vi "Kxx_Kxy_B_cs580 _KEguard2.vi"() -> ()   [LabVIEW 2023]
uses:
  <instrlib>/Keithley 622x LV 2009/Utility/Typedefs/KE622x -- Instrument Type.ctl
  Typedefs/Kxx_Kxy_state_machine_cases.ctl
  Z:/Labview Control Software/Keithley 622x LV 2009/Typedefs/KE622x -- On Off Control.ctl
  Z:/Labview Control Software/Keithley 622x LV 2009/Configure/Output/Typedefs/KE6221 -- Output Response.ctl
  Z:/Labview Control Software/Keithley 622x LV 2009/Configure/Source/Typedefs/KE622x -- Voltage Limit.ctl
  <vilib>/Analysis/1siggen.llb/Ramp Pattern by Samples.vi
  <vilib>/Analysis/baseanly.llb/Mean (DBL).vi
  <vilib>/Instr/_visa.llb/VISA Configure Serial Port (Instr).vi
  <vilib>/Utility/file.llb/Write To Spreadsheet File (string).vi
  MQM Data Transfer All.vi
  <vilib>/Utility/file.llb/Read Delimited Spreadsheet (DBL).vi
  Global Variables/Thermometers.vi
  <instrlib>/Keithley 622x LV 2009/Keithley 622x.lvlib
  <vilib>/Analysis/NI_AALBase.lvlib
  Drivers/Keithley 2182/Keithley 2182.lvlib
panel:
  in  "Kxy data":dbl[](array[numeric])
  in  "Kxx data":dbl[](array[numeric])
  in  "T_avg data":dbl[](array[numeric])
  in  "dTxx":dbl
  in  "HTR Power":dbl
  in  "dTxy":dbl
  in  "T_avg":dbl
  in  "T_H Array":dbl[](array[numeric])
  in  "T_C1 Array":dbl[](array[numeric])
  in  "T_C2 Array":dbl[](array[numeric])
  in  "HTR Voltage Array":dbl[](array[numeric])
  in  "?":enum32{"Setup", "Plotting", "Error Readouts"}(tab)
  in  "DeltaT (fraction of tsp)":dbl=0.05
  in  "Sample_t":dbl
  in  "Sample_w":dbl
  in  "Sample_Lxx":dbl
  in  "Heater Current File (H, T, current)":path
  out "Heater Current \nArray":dbl[](array[numeric])
  out "Ramp Pattern":dbl[](array[numeric])
  in  "Tstart (K)":dbl=3.0
  in  "Tend (K)":dbl=4.0
  in  "Steps":i16=2
  in  "Log (on)\nLin (off) (Temperature setpoints)":bool=TRUE
  in  "Initial Heater Current (A)":dbl=1e-06
  in  "Hstart (Oe)":dbl
  in  "Hend (Oe)":dbl
  in  "Field Steps":i16=1
  in  "Log (on)\nLin (off)  (Field setpoints)":bool
  in  "Sample_Lxy":dbl=0.0005
  in  "Test?":bool
  in  "Calibration Only?":bool
  in  "Exchange gas?":bool
  in  "Preset Heater Current Array?":bool
  in  "T Current Source":refnum<visa-resource-name>="6221B"
  in  "HTR Current Source":refnum<visa-resource-name>="CS580-1"
  in  "DC Voltmeter":refnum<visa-resource-name>="2182"
  in  "Thermometer Frequency (Hz)":string="37"
  in  "Initial Thermometer Current (A)":string="1.4142e-7"
  in  "Final Field (Oe)":dbl
  in  "Final Temperature (K)":dbl=1.7
  in  "Filename":path=path "C:/User Data/Luke/Kxx/NaYSe2/NaYSe2_1p7_100K_log_100_9T_8_23_21"
  in  "Heater Only?":bool
  in  "Running avg size":dbl=500.0 format="%#_13g"
  in  "std/mean thresh":dbl=1e-05 format="%#_13g"
  in  "slope/mean thresh":dbl=1e-07 format="%#_13g"
  in  "Guard HTR Current Source":refnum<visa-resource-name>
  in  "HTR Guard Current Factor":dbl
  out "Kxx Plot":cluster{dbl[], dbl[]}(graph)
  out "Kxy Plot":cluster{dbl[], dbl[]}(graph)
  out "All Data":cluster{dbl[], dbl[]}[](graph)
  in  "Finish":bool
  out "Data Rate (ms)":u32
  in  "Delay (ms)":dbl=300.0
  in  "Quick Data Recording":bool=TRUE
  out "Tsp":dbl
  out "HTR_Current":dbl
  out "Mask":dbl
  out "HTR_Voltage":dbl
  out "T_H":dbl
  out "T_C1":dbl
  out "I_therm":dbl
  out "T_C2":dbl
  in  "Display Elements":cluster{"X":bool, "Y":bool, "Name":u16}[](array[cluster]) {"Name" items=["Time (ms)", "Temperature (K)", "Field (T)", "LI_1_X", "LI_1_theta", "LI_2_X", "LI_2_theta", "LI_3_X", "LI_3_theta", "DC_V", "DC_I", "mask", "tsp", "I_therm", "T_H", "T_C1", "T_C2", "Fieldsp"]}
  in  "X-Axis":u16(ring) items=["Linear", "Reciprocal", "Log10"]
  in  "Y-Axis":u16(ring) items=["Linear", "Reciprocal", "Log10"]
  out "Fieldsp":dbl
  out "Global Stop":bool
  out "Thermometers":cluster{"T_H":dbl, "T_C1":dbl, "T_C2":dbl}
  out "QD error out":errorcluster
  out "KE6221 error out":errorcluster
  out "KE2182 error out":errorcluster
  out "Guard Heater Error":errorcluster
  # "TURN ON HIGH VACUUM!"
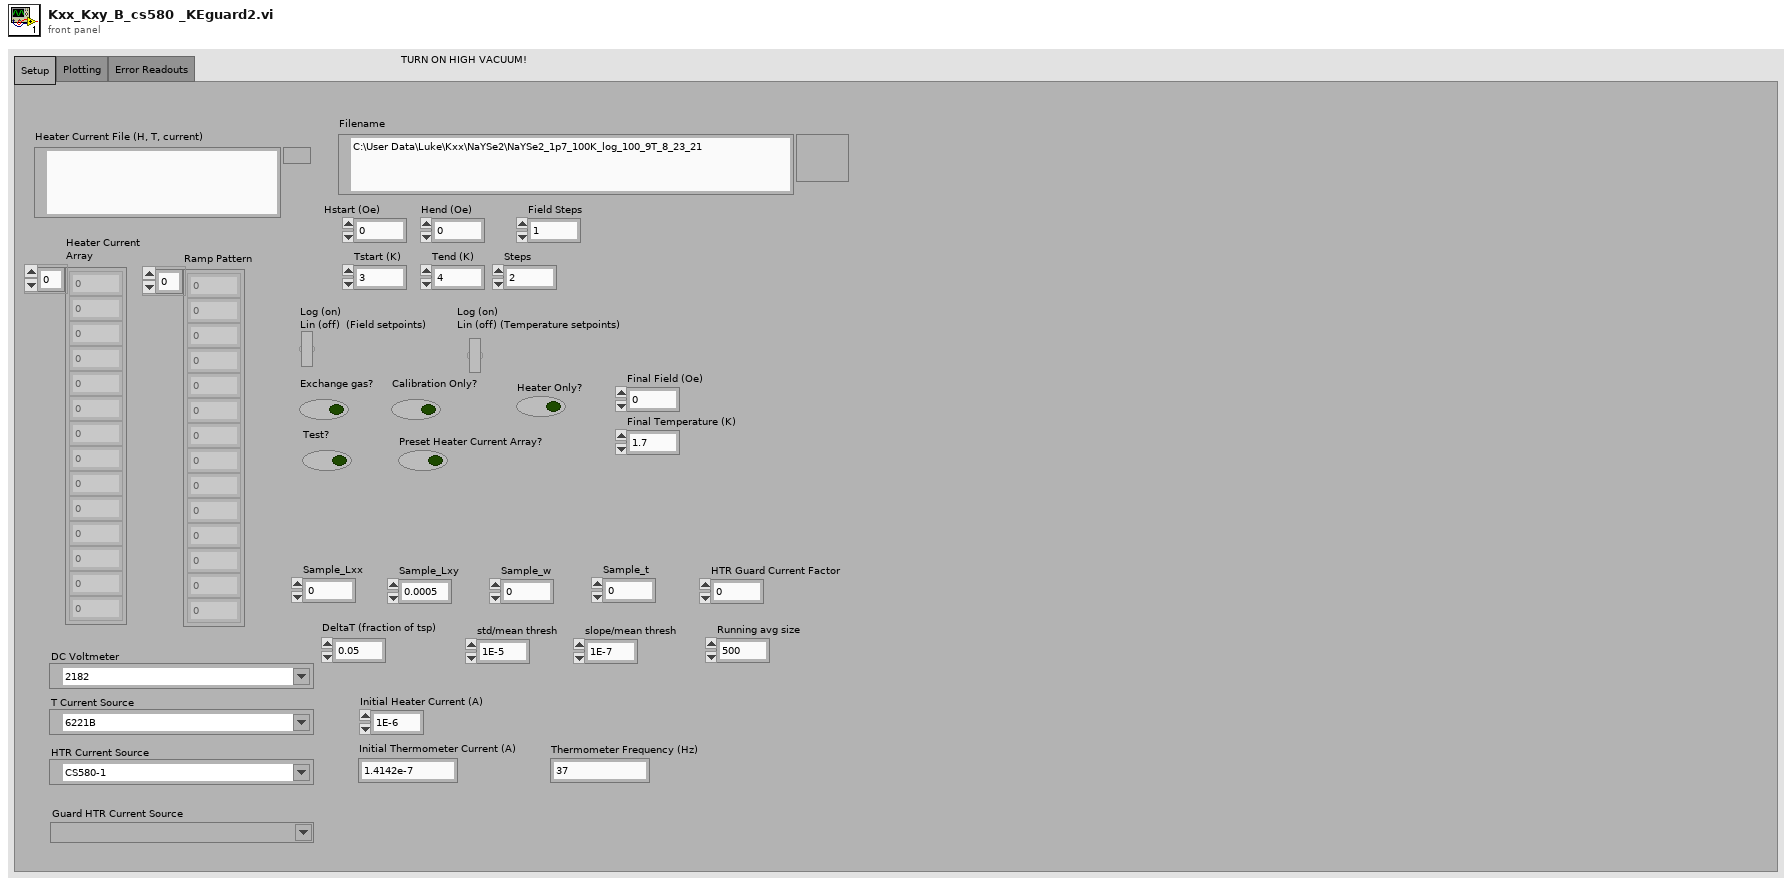
[diagram p1: front panel]
types:
  T1 = typedef "Keithley 622x.lvlib/KE622x -- Instrument Type.ctl" = enum16{"KE6220", "KE6221"}
  T2 = typedef "Kxx_Kxy_state_machine_cases.ctl" = enum16{"Initialize", "Wait to Stabilize (no heat)", "Measure (no heat)", "Turn on Heater, stabilize", "Measure (heat)", "Turn off Heater", "Assign Heater Current", "Plot", "End"}
  T3 = typedef "Keithley 622x.lvlib/KE622x -- Voltage Limit.ctl" = dbl
  T4 = typedef "Keithley 622x.lvlib/KE6221 -- Output Response.ctl" = enum16{"Fast", "Slow"}
  T5 = typedef "Keithley 622x.lvlib/KE622x -- On Off Control.ctl" = enum16{"Off", "On"}
  T6 = cluster{"T_avg data":dbl[], "Kxx data":dbl[], "Kxy data":dbl[]}
  T7 = cluster{"T_avg":dbl, "dTxx":dbl, "dTxy":dbl, "HTR Power":dbl, "HTR Voltage Array":dbl[], "T_H Array":dbl[], "T_C1 Array":dbl[], "T_C2 Array":dbl[], "error out":errorcluster}
  T8 = typedef "ZI_Frontpanel_All.ctl" = cluster{"Lockin 1 Demod 0":cluster{"R(V)":dbl, "Theta (deg)":dbl, "Timestamp (ms)":u32, "X(V)":dbl, "Y(V)":dbl, "frequency (Hz)":dbl, "output voltage (V)":dbl}, "Lockin 2 Demod 0":cluster{"R(V)":dbl, "Theta (deg)":dbl, "Timestamp (ms)":u32, "X(V)":dbl, "Y(V)":dbl, "frequency (Hz)":dbl, "output voltage (V)":dbl}, "Lockin 3 Demod 0":cluster{"R(V)":dbl, "Theta (deg)":dbl, "Timestamp (ms)":u32, "X(V)":dbl, "Y(V)":dbl, "frequency (Hz)":dbl, "output voltage (V)":dbl}, "Lockin 4 Demod 0":cluster{"R(V)":dbl, "Theta (deg)":dbl, "Timestamp (ms)":u32, "X(V)":dbl, "Y(V)":dbl, "frequency (Hz)":dbl, "output voltage (V)":dbl}, "LI1 active":bool, "LI2 active":bool, "LI3 active":bool, "LI4 active":bool}
  T9 = typedef "PPMS_Status.ctl" = cluster{"Field":cluster{"Field (T)":dbl, "Field stable":bool, "Timestamp (ms)":u32}, "Temperature":cluster{"Temperature (K)":dbl, "Temperature stable":bool, "Timestamp (ms)":u32}}
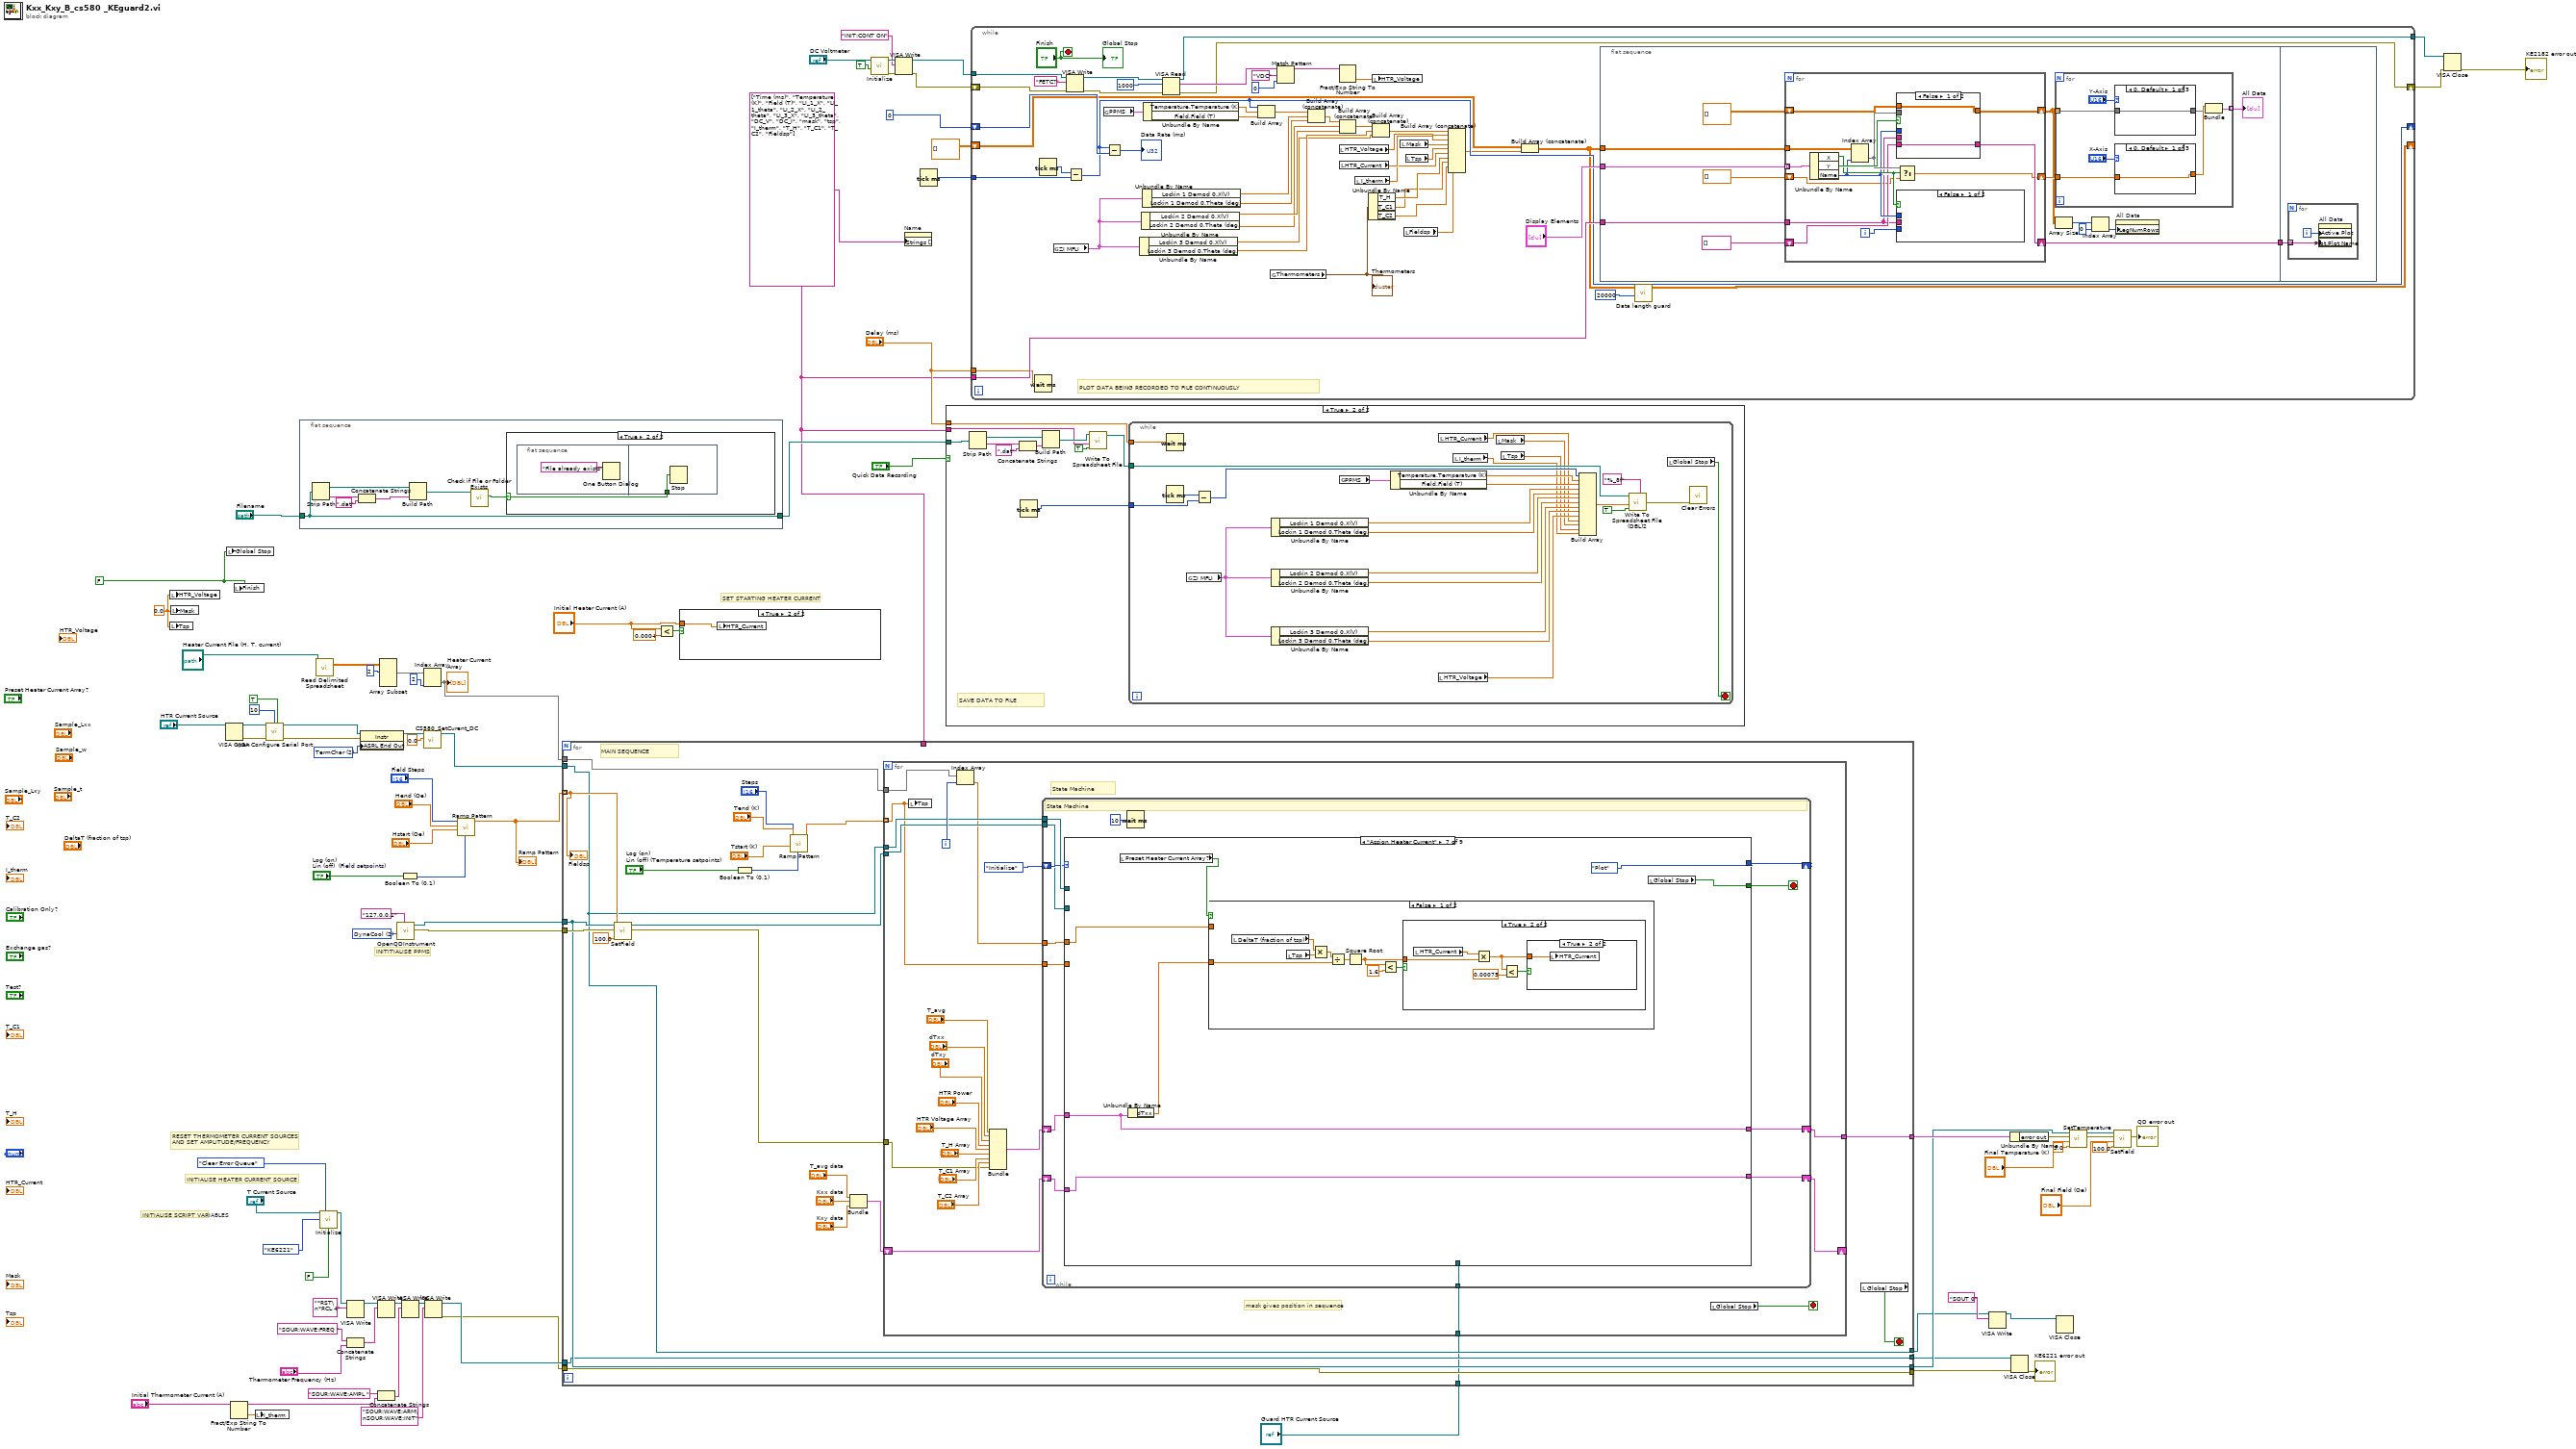
[diagram p0: block diagram]
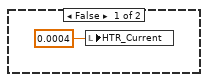
[diagram p2: hidden frame]
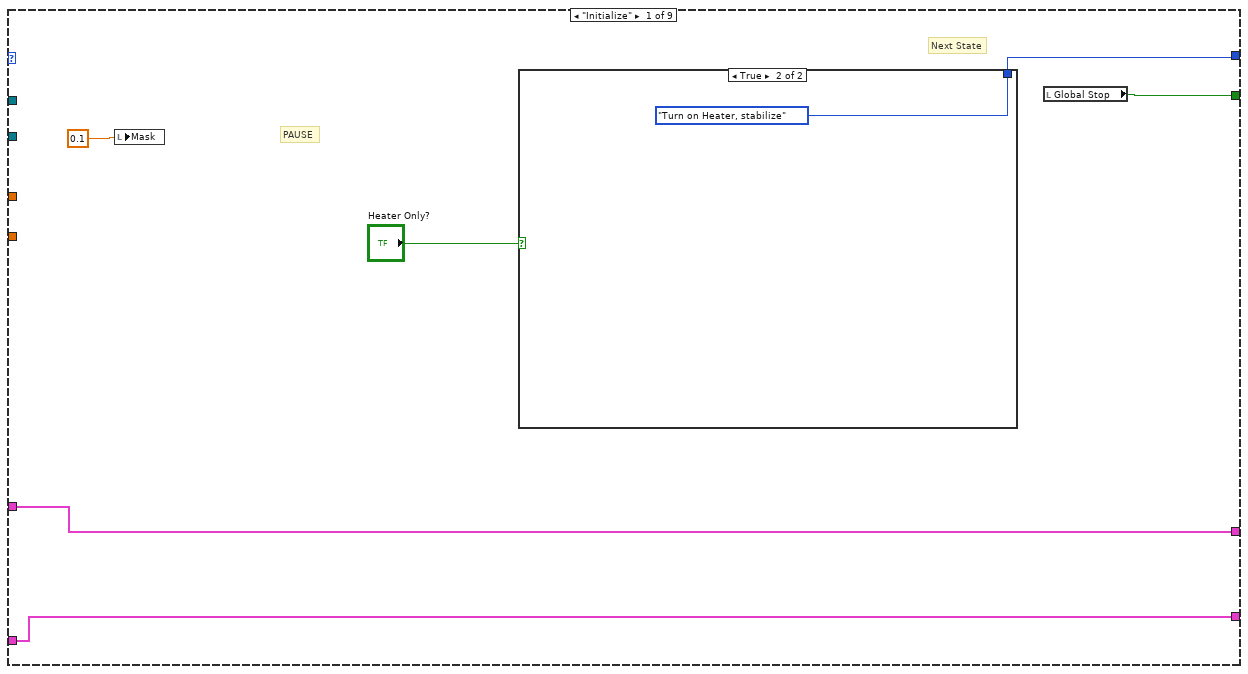
[diagram p4: hidden frame]
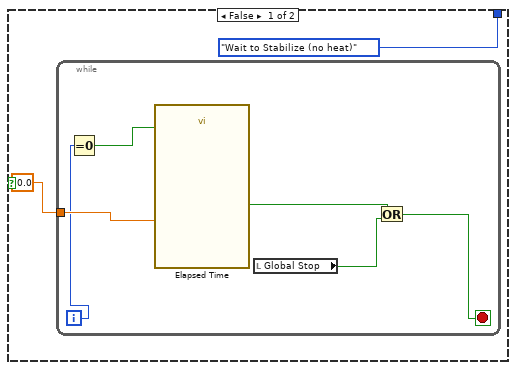
[diagram p5: hidden frame]
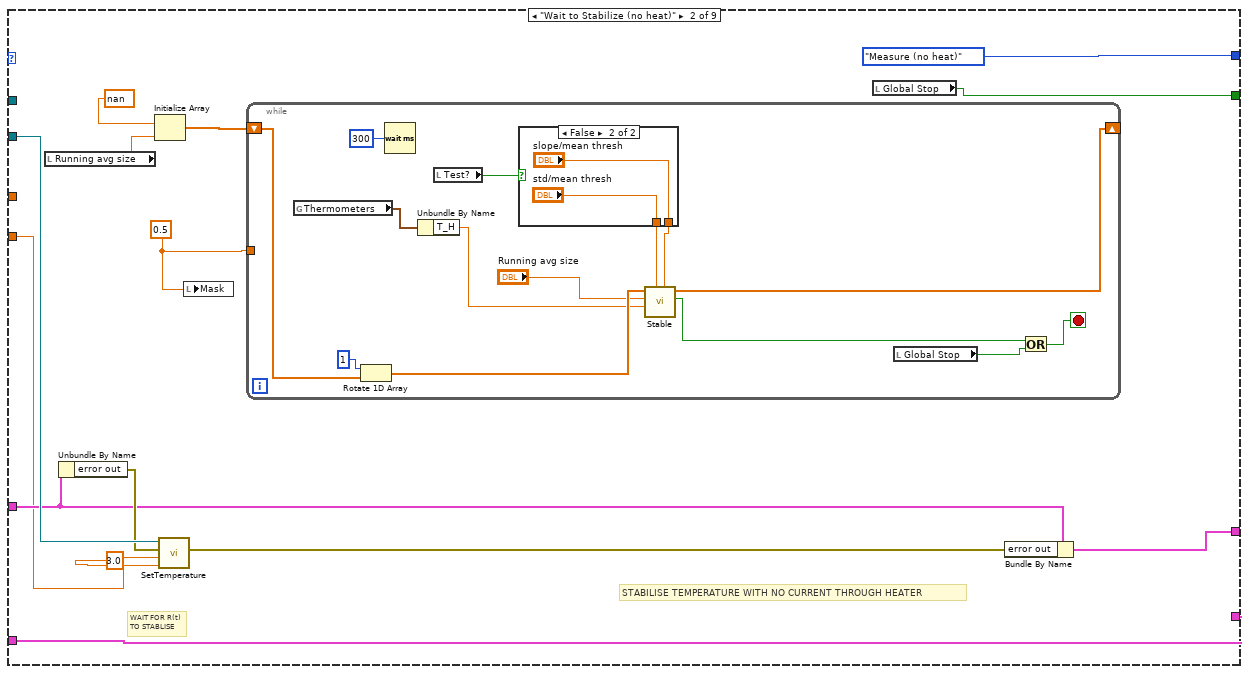
[diagram p6: hidden frame]
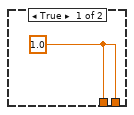
[diagram p7: hidden frame]
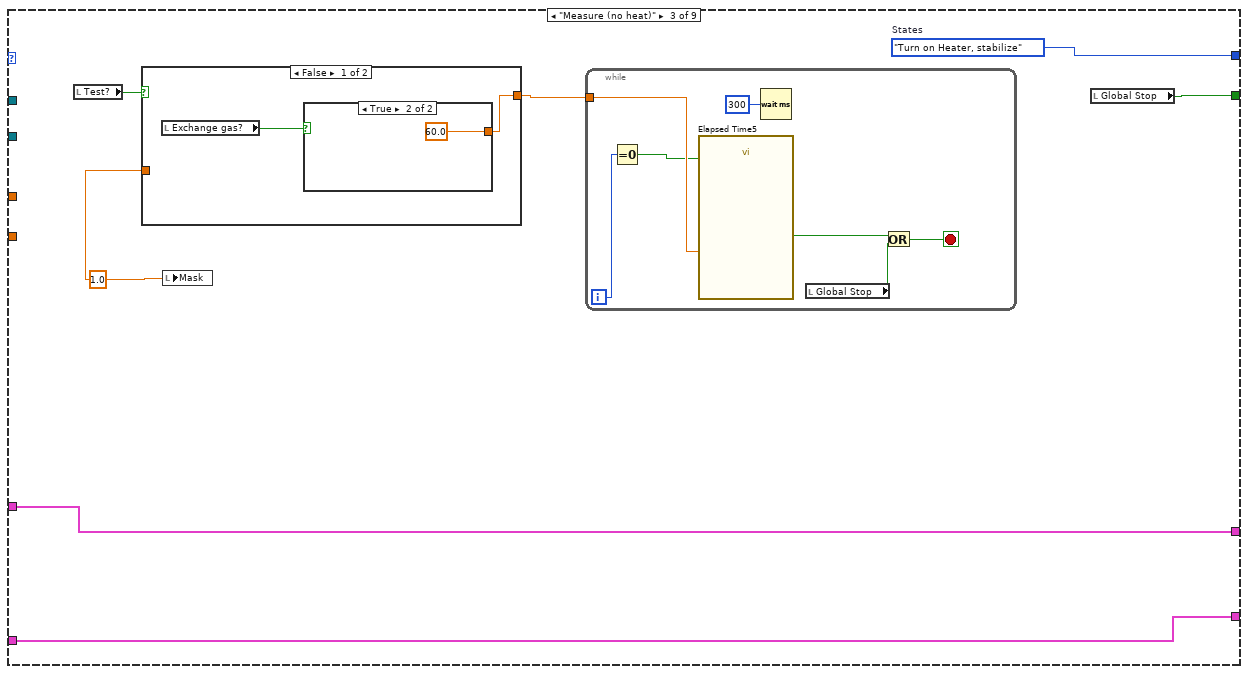
[diagram p8: hidden frame]
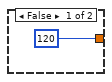
[diagram p9: hidden frame]
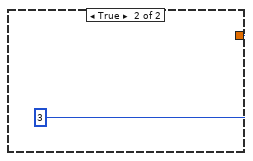
[diagram p10: hidden frame]
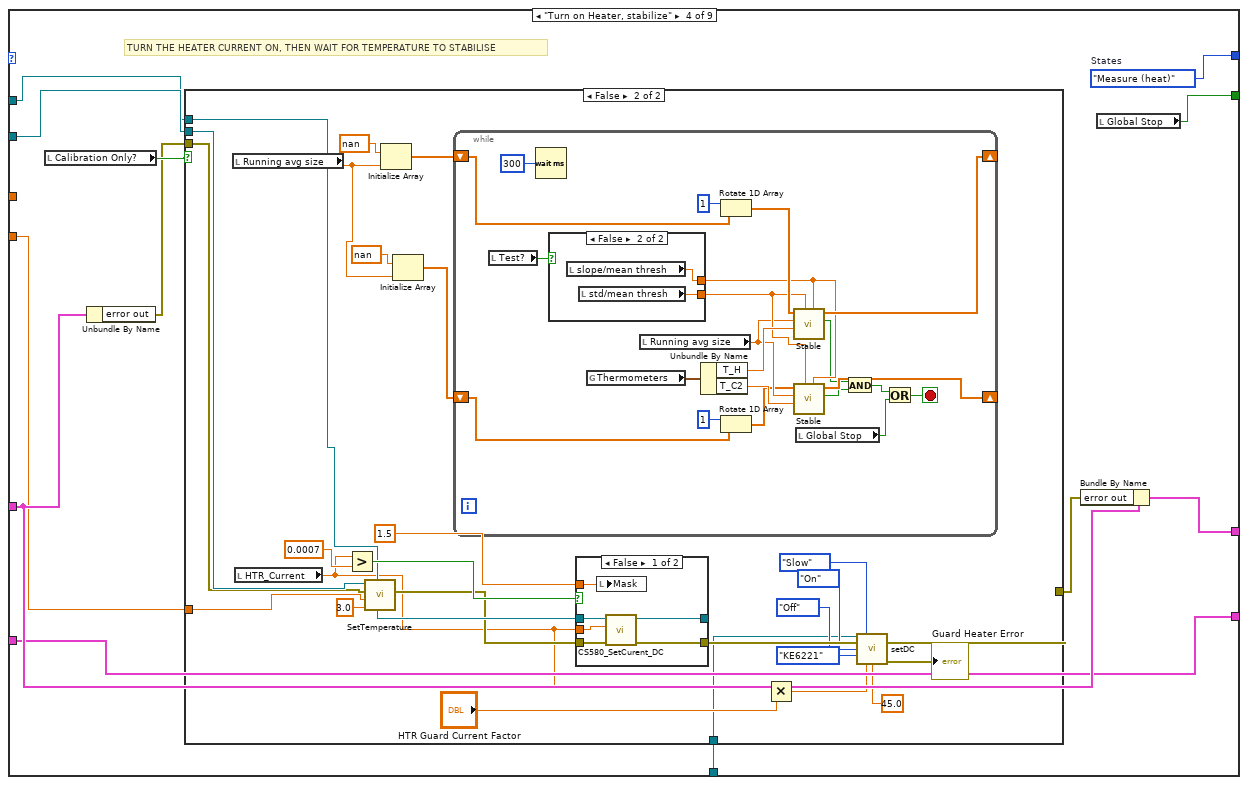
[diagram p11: hidden frame]
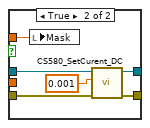
[diagram p13: hidden frame]
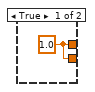
[diagram p14: hidden frame]
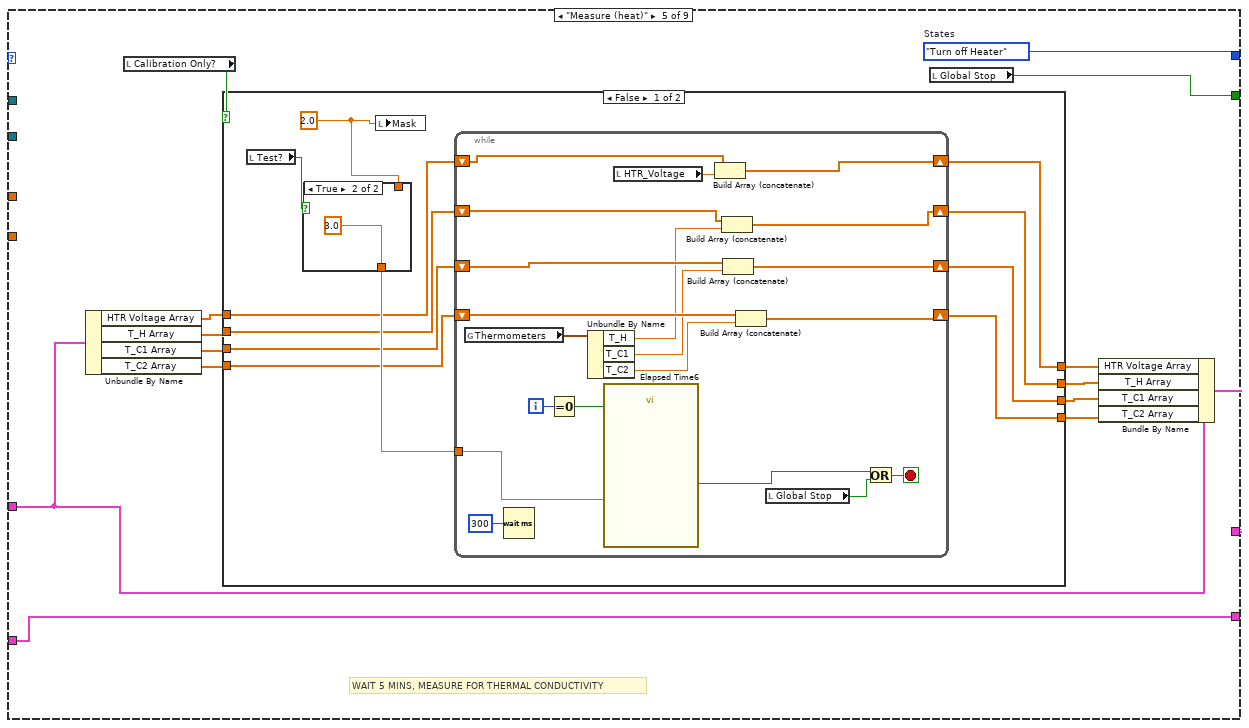
[diagram p15: hidden frame]
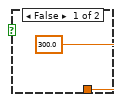
[diagram p16: hidden frame]
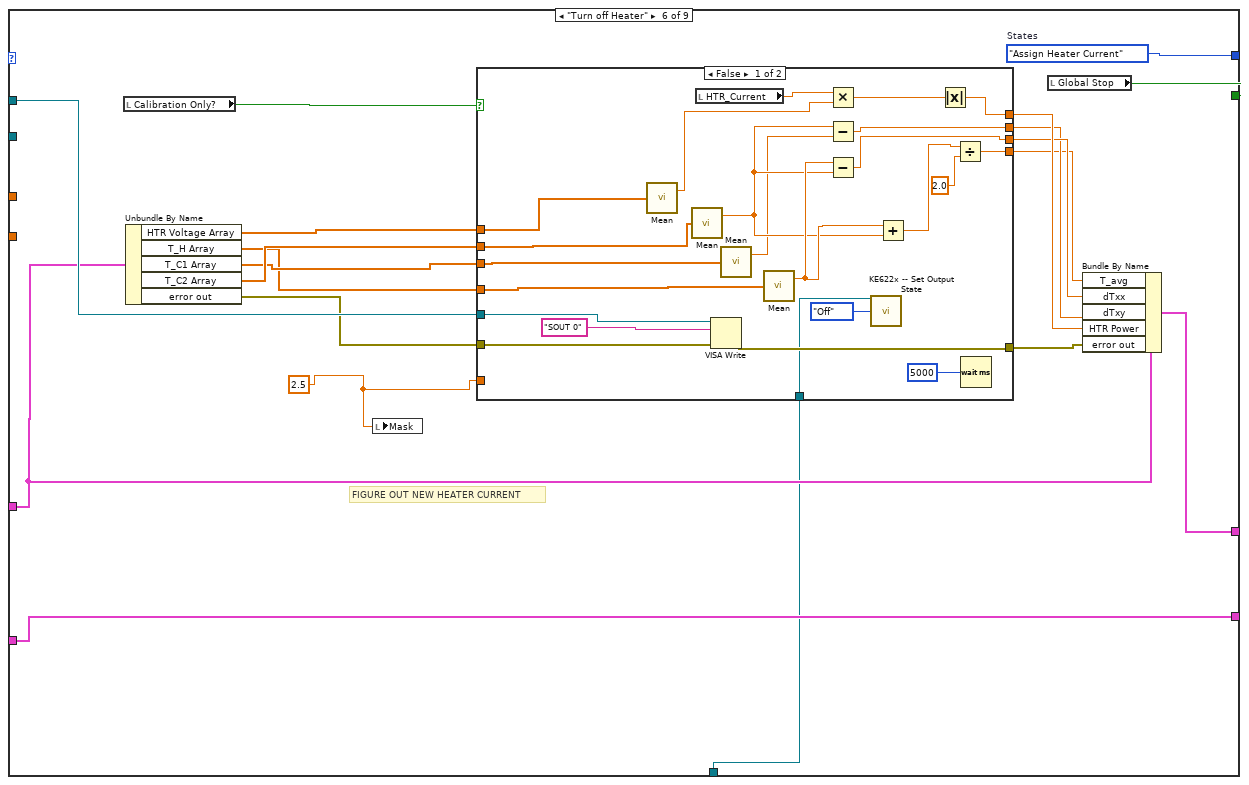
[diagram p18: hidden frame]
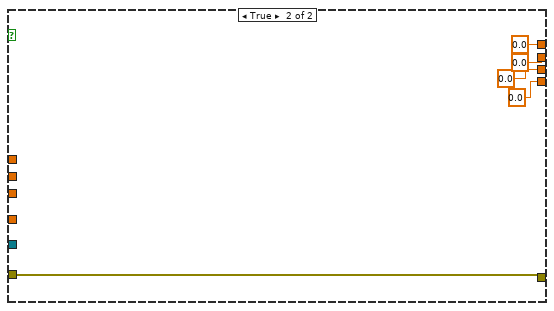
[diagram p19: hidden frame]
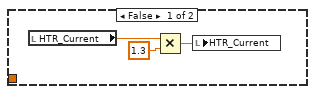
[diagram p20: hidden frame]
diagram:
  w7 = FALSE ("Calibration confirmed")
  w6 = string[] ["Time (ms)", "Temperature (K)", "Field (T)", "LI_1_X", "LI_1_theta", "LI_2_X", "LI_2_theta", "LI_3_X", "LI_3_theta", "DC_V", "DC_I", "mask", "tsp", "I_therm", "T_H", "T_C1", "T_C2", "Fieldsp"] ("element")
  w57 = u16 2 items=["None", "Last Bit", "TermChar", "Break"] ("Serial Settings:End Mode for Writes")
  w75 = 0.0 ("Mask")
  w82 = 2 items=["PPMS", "VersaLab", "DynaCool", "SVSM"] ("Instrument Type")
  # "SET STARTING HEATER CURRENT"
  # "INITIALISE HEATER CURRENT SOURCE"
  # "RESET THERMOMETER CURRENT SOURCES\nAND SET AMPLITUDE/FREQUENCY"
  # "INITITIALISE PPMS"
  # "INITIALISE SCRIPT VARIABLES"
  n1 = local write "HTR_Voltage"(w75) -> ()
  n2 = local write "Tsp"(w75) -> ()
  n3 = local write "Mask"(w75) -> ()
  n4 = VISA Open(VISA resource name="HTR Current Source") -> (VISA resource name=w53:refnum<visa-resource-name>, error out=w54:errorcluster)  [unwired: 4 in]
  n5 = local write "Global Stop"(w7) -> ()
  n6 = Fract/Exp String To Number(string="Initial Thermometer Current (A)") -> (number=w65:dbl)  [unwired: 3 in, 1 out]
  n7 = local write "Finish"(w7) -> ()
  n8 = local write "I_therm"(w65) -> ()
  n9 = call-poly "VISA Configure Serial Port"("VISA resource name"=w53, "termination char\n(0xA = '\\n' = LF)"=u8 10 ("termination char\n(0xA = '\\n' = LF)"), "Enable Termination\nChar (T)"=TRUE ("Enable Termination\nChar (T)"), "error in (no error)"=w54) -> ("VISA resource name out"=w55:refnum<visa-resource-name>, "error out"=w56:errorcluster)  [unwired: 10 in]
  n10 = flat-sequence {
    tunnel: "Filename" -> [w89]
    tunnel: [w89] -> w26
    frame #0 {
      n11 = Strip Path(path=w89) -> (stripped path=w93:path, name=w90:string)
      n12 = Concatenate Strings(w90, ".dat") -> (w92:string)
      n13 = Build Path(base path=w93, name or relative path=w92) -> (appended path=w88:path)
      n14 = call <vilib>:"Check if File or Folder Exists.vi"("path"=w88) -> ("file or folder exists?"=w87:bool)  [unwired: 8 in, 2 out]
      n15 = case shown="True" w87 {
        selector: w87 -> [_ w94]
        frame False {
        }
        frame True {
          n16 = flat-sequence {
            tunnel: w94 -> [w96]
            frame #0 {
              n17 = One Button Dialog(message="File already exists") -> ()  [unwired: 1 in, 1 out]
            }
            frame #1 {
              n18 = Stop(stop? (T)=w96) -> ()
            }
          }
        }
      }
    }
  }
  n19 = call-poly <vilib>:"Read Delimited Spreadsheet.vi"("file path (dialog if empty)"="Heater Current File (H, T, current)") -> ("all rows"=w48:dbl[][])  [unwired: 9 in, 5 out]
  n20 = call <instrlib>:"Initialize.vi"("VISA resource name"="T Current Source", "Error Queue Option"=enum16{"Clear Error Queue", "Error Query"}."Clear Error Queue", "Instrument Type"=KE622x_--_Instrument_Type."KE6221", "Reset? (T)"=FALSE) -> ("VISA resource name out"=w73:refnum<visa-resource-name>)  [unwired: 10 in, 1 out]
  n21 = VISA Write(VISA resource name=w73, write buffer="*RST\n*RCL 4") -> (VISA resource name out=w67:refnum<visa-resource-name>)  [unwired: 1 in, 2 out]
  n22 = Concatenate Strings("SOUR:WAVE:FREQ " ("string"), "Thermometer Frequency (Hz)") -> (w72:string)
  n23 = property class="Instr"(reference=w55, error in=w56, "ASRL End Out"=w57) -> (reference out=w51:refnum<visa-resource-name>)  [unwired: 1 out]
  n24 = VISA Write(VISA resource name=w67, write buffer=w72) -> (VISA resource name out=w66:refnum<visa-resource-name>)  [unwired: 1 in, 2 out]
  n25 = Concatenate Strings("SOUR:WAVE:AMPL " ("string"), "Initial Thermometer Current (A)") -> (w69:string)
  n26 = Array Subset(array=w48, index (row)=2 ("index")) -> (w46:dbl[][])  [unwired: 3 in]
  n27 = call <instrlib>:"OpenQDInstrument.vi"("IP Address"="127.0.0.1", "Instrument Type"=w82) -> ("error out"=w25:errorcluster, "Instrument Ref"=w23:refnum<k24>)  [unwired: 6 in]
  n28 = VISA Write(VISA resource name=w66, write buffer=w69) -> (VISA resource name out=w43:refnum<visa-resource-name>)  [unwired: 1 in, 2 out]
  n29 = Boolean To (0,1)(Boolean="Log (on)\nLin (off)  (Field setpoints)") -> (0, 1=w60:i16)
  n30 = Index Array(array=w46, index (col)=2 ("disabled index (col)")) -> (element=w41:dbl[])  [unwired: 1 in]
  "Heater Current \nArray" <- w41
  n31 = call "CS580_SetCurent_DC.vi"("Current (A)"=0.0, "VISA Refnum in"=w51) -> ("VISA resource name out"=w24:refnum<visa-resource-name>)  [unwired: 8 in, 1 out]
  n32 = VISA Write(VISA resource name=w43, write buffer="SOUR:WAVE:ARM\nSOUR:WAVE:INIT") -> (VISA resource name out=w16:refnum<visa-resource-name>, error out=w12:errorcluster)  [unwired: 1 in, 1 out]
  n33 = call-poly <vilib>:"Ramp Pattern.vi"("type"=w60, "start"="Hstart (Oe)", "end"="Hend (Oe)", "samples"="Field Steps") -> ("Ramp Pattern"=w42:dbl[])  [unwired: 6 in, 1 out]
  "Ramp Pattern" <- w42
  n34 = for {
    tunnel: w42 -> [w119] mode=indexing
    tunnel: w23 -> [w102]
    tunnel: w25 -> [w117]
    tunnel: w41 -> [w110]
    tunnel: w24 -> [w98]
    tunnel: [w103] -> w18
    tunnel: w16 -> [w101]
    tunnel: [w102] -> w15
    tunnel: [w101] -> w14
    tunnel: w12 -> [w100]
    tunnel: [w100] -> w11
    tunnel: [w98] -> w4
    tunnel: w6 -> [_]
    tunnel: "Guard HTR Current Source" -> [w97]
    stop <- w99 stop-if-true
    # "MAIN SEQUENCE"
    n35 = call <instrlib>:"SetField.vi"("Rate"=100.0, "Field"=w119, "error in (no error)"=w117, "Instrument Ref In"=w102) -> ("error out"=w109:errorcluster, "Instrument Ref Out"=w108:refnum<k24>)  [unwired: 3 in, 1 out]
    n36 = Boolean To (0,1)(Boolean="Log (on)\nLin (off) (Temperature setpoints)") -> (0, 1=w114:i16)
    n37 = call-poly <vilib>:"Ramp Pattern.vi"("type"=w114, "start"="Tstart (K)", "end"="Tend (K)", "samples"="Steps") -> ("Ramp Pattern"=w116:dbl[])  [unwired: 6 in, 1 out]
    n38 = Bundle("T_avg data"="T_avg data", "Kxx data"="Kxx data", "Kxy data"="Kxy data") -> (w104:T6)  [unwired: 1 in]
    n39 = for {
      tunnel: w116 -> [w123] mode=indexing
      tunnel: w110 -> [w141]
      tunnel: w109 -> [w128]
      tunnel: w98 -> [w138]
      tunnel: w108 -> [w137]
      shift-right: [w122] -> _
      shift-left: w104 -> [w121]
      tunnel: [w125] -> w103
      tunnel: w97 -> [w120]
      i -> [w140]
      stop <- w124 stop-if-true
      # "State Machine"
      # "mask gives position in sequence"
      n40 = local write "Tsp"(w123) -> ()
      n41 = Index Array(array=w141, index=w140) -> (element=w126:dbl)
      n42 = Bundle("T_avg"="T_avg", "dTxx"="dTxx", "dTxy"="dTxy", "HTR Power"="HTR Power", "HTR Voltage Array"="HTR Voltage Array", "T_H Array"="T_H Array", "T_C1 Array"="T_C1 Array", "T_C2 Array"="T_C2 Array", "error out"=w128) -> (w127:T7)  [unwired: 1 in]
      n43 = while {
        shift-right: [w154] -> _
        shift-left: Kxx_Kxy_state_machine_cases."Initialize" -> [w151]
        tunnel: w138 -> [w152]
        tunnel: w137 -> [w147]
        shift-right: [w150] -> w125
        shift-left: w127 -> [w149]
        tunnel: w126 -> [w148]
        tunnel: w123 -> [w145]
        shift-right: [w144] -> w122
        shift-left: w121 -> [w143]
        tunnel: w120 -> [w142]
        stop <- w146 stop-if-true
        # "State Machine"
        n44 = case shown="\"Assign Heater Current\"" w151 {
          selector: w151 -> [_ _ _ _ _ _ _ _ w447]
          tunnel: w147 -> [_ w179 _ w230 _ _ _ _ _]
          tunnel: [w159 Kxx_Kxy_state_machine_cases."Measure (no heat)" w205 w228 w306 w361 Kxx_Kxy_state_machine_cases."Plot" w435 w447] -> w154
          tunnel: w152 -> [_ _ _ w229 _ w362 _ _ _]
          tunnel: [w158 w175 w204 w224 w297 w349 w396 w434 w446] -> w150
          tunnel: w149 -> [w158 w176 w204 w226 w296 w356 w396 w434 w446]
          tunnel: w143 -> [w157 w174 w203 w223 w295 w348 w395 w425 w445]
          tunnel: [w157 w174 w203 w223 w295 w348 w395 w421 w445] -> w144
          tunnel: w148 -> [_ _ _ _ _ _ w394 _ _]
          tunnel: [w156 w173 w202 w222 w294 w347 w393 w418 TRUE] -> w146
          tunnel: w145 -> [_ w172 _ w221 _ _ _ _ _]
          tunnel: w142 -> [_ _ _ w220 _ w345 _ _ _]
          frame "Initialize" {
            # "Next State"
            # "PAUSE"
            n45 = local write "Mask"(0.1 ("Mask")) -> ()
            n46 = case shown="True" "Heater Only?" {
              tunnel: [Kxx_Kxy_state_machine_cases."Wait to Stabilize (no heat)" Kxx_Kxy_state_machine_cases."Turn on Heater, stabilize"] -> w159
              frame False {
                n47 = while {
                  tunnel: 10.0 ("Time Target (s)") -> [w168]
                  i -> [w164]
                  stop <- w165 stop-if-true
                  n48 = Equal To 0?(x=w164) -> (x = 0?=w163:bool)
                  n49 = call "Elapsed Time"("Time Target (s)"=w168, "Reset"=w163) -> ("Time has Elapsed"=w167:bool)  [unwired: 10 in, 7 out]
                  n50 = local read "Global Stop"() -> (w166:bool)
                  n51 = Or(x=w167, y=w166) -> (x .or. y?=w165:bool)
                }
              }
              frame True {
              }
            }
            n52 = local read "Global Stop"() -> (w156:bool)
          }
          frame "Wait to Stabilize (no heat)" {
            w170 = 0.5 ("Mask")
            # "STABILISE TEMPERATURE WITH NO CURRENT THROUGH HEATER"
            # "WAIT FOR R(t)\nTO STABLISE"
            n53 = local read "Running avg size"() -> (w181:dbl)
            n54 = Unbundle By Name(w176) -> ("error out"=w177:errorcluster)
            n55 = Initialize Array(nan ("Element"), w181) -> (w183:dbl[])
            n56 = call <instrlib>:"SetTemperature.vi"("Rate"=3.0, "Temperature"=w172, "error in (no error)"=w177, "Instrument Ref In"=w179) -> ("error out"=w171:errorcluster)  [unwired: 3 in, 2 out]
            n57 = local write "Mask"(w170) -> ()
            n58 = while {
              shift-right: [w186] -> _
              shift-left: w183 -> [w196]
              tunnel: w170 -> [_]
              stop <- w192 stop-if-true
              n59 = global read "Thermometers.vi" "Thermometers"() -> (w191:cluster{"T_H":dbl, "T_C1":dbl, "T_C2":dbl})
              n60 = Rotate 1D Array(1:w196, 2:1 ("n")) -> (0:w190:dbl[])
              n61 = Wait (ms)(milliseconds to wait=u32 300) -> ()  [unwired: 1 out]
              n62 = Unbundle By Name(w191) -> ("T_H"=w188:dbl)
              n63 = local read "Test?"() -> (w194:bool)
              n64 = case shown="False" w194 {
                tunnel: [w198 "slope/mean thresh"] -> w187
                tunnel: [w198 "std/mean thresh"] -> w184
                frame True {
                  w198 = 1.0 ("y")
                }
                frame False {
                }
              }
              n65 = call "Stable.vi"("slope/mean thresh"=w187, "std/mean thresh"=w184, "New data point"=w188, "Number of points"="Running avg size", "Array in"=w190) -> ("Stable?"=w185:bool, "Array out"=w186:dbl[])  [unwired: 5 in]
              n66 = local read "Global Stop"() -> (w193:bool)
              n67 = Or(x=w185, y=w193) -> (x .or. y?=w192:bool)
            }
            n68 = local read "Global Stop"() -> (w173:bool)
            n69 = Bundle By Name(cluster=w176, "error out"=w171) -> (w175:T7)
          }
          frame "Measure (no heat)" {
            w205 = Kxx_Kxy_state_machine_cases."Turn on Heater, stabilize"  # States
            w201 = 1.0 ("Mask")
            n70 = local read "Test?"() -> (w207:bool)
            n71 = case shown="False" w207 {
              tunnel: [w208 u32 3 ("milliseconds to wait")] -> w206
              tunnel: w201 -> [_ _]
              frame False {
                n72 = local read "Exchange gas?"() -> (w209:bool)
                n73 = case shown="True" w209 {
                  tunnel: [120 60.0 ("Time to Wait (s)")] -> w208
                  frame False {
                  }
                  frame True {
                  }
                }
              }
              frame True {
              }
            }
            n74 = local write "Mask"(w201) -> ()
            n75 = while {
              tunnel: w206 -> [w217]
              i -> [w214]
              stop <- w216 stop-if-true
              n76 = Equal To 0?(x=w214) -> (x = 0?=w213:bool)
              n77 = call "Elapsed Time5"("Time Target (s)"=w217, "Reset"=w213) -> ("Time has Elapsed"=w215:bool)  [unwired: 10 in, 7 out]
              n78 = Wait (ms)(milliseconds to wait=u32 300) -> ()  [unwired: 1 out]
              n79 = local read "Global Stop"() -> (w219:bool)
              n80 = Or(x=w215, y=w219) -> (x .or. y?=w216:bool)
            }
            n81 = local read "Global Stop"() -> (w202:bool)
          }
          frame "Turn on Heater, stabilize" {
            w228 = Kxx_Kxy_state_machine_cases."Measure (heat)"  # States
            # "TURN THE HEATER CURRENT ON, THEN WAIT FOR TEMPERATURE TO STABILISE"
            n82 = local read "Calibration Only?"() -> (w231:bool)
            n83 = Unbundle By Name(w226) -> ("error out"=w227:errorcluster)
            n84 = case shown="False" w231 {
              tunnel: w230 -> [_ w257]
              tunnel: w227 -> [w232 w250]
              tunnel: [w232 w251] -> w225
              tunnel: w229 -> [_ w252]
              tunnel: w221 -> [_ w247]
              tunnel: w220 -> [_ w233]
              frame True {
              }
              frame False {
                n85 = local read "Running avg size"() -> (w243:dbl)
                n86 = local read "HTR_Current"() -> (w235:dbl)
                n87 = Greater?(x=w235, y=0.0007) -> (0:w253:bool)
                n88 = call <instrlib>:"SetTemperature.vi"("Rate"=3.0, "Temperature"=w247, "error in (no error)"=w250, "Instrument Ref In"=w257) -> ("error out"=w249:errorcluster)  [unwired: 3 in, 2 out]
                n89 = Initialize Array(nan ("Element"), w243) -> (w256:dbl[])
                n90 = Initialize Array(nan ("Element"), w243) -> (w244:dbl[])
                n91 = while {
                  shift-right: [w287] -> _
                  shift-left: w256 -> [w289]
                  shift-right: [w273] -> _
                  shift-left: w244 -> [w276]
                  stop <- w285 stop-if-true
                  n92 = local read "Test?"() -> (w286:bool)
                  n93 = Wait (ms)(milliseconds to wait=u32 300) -> ()  [unwired: 1 out]
                  n94 = case shown="False" w286 {
                    tunnel: [w291 w293] -> w280
                    tunnel: [w291 w292] -> w279
                    frame True {
                      w291 = 1.0 ("y")
                    }
                    frame False {
                      n95 = local read "slope/mean thresh"() -> (w293:dbl)
                      n96 = local read "std/mean thresh"() -> (w292:dbl)
                    }
                  }
                  n97 = global read "Thermometers.vi" "Thermometers"() -> (w283:cluster{"T_H":dbl, "T_C1":dbl, "T_C2":dbl})
                  n98 = local read "Running avg size"() -> (w278:dbl)
                  n99 = Unbundle By Name(w283) -> ("T_H"=w281:dbl, "T_C2"=w277:dbl)
                  n100 = Rotate 1D Array(1:w289, 2:1 ("n")) -> (0:w282:dbl[])
                  n101 = Rotate 1D Array(1:w276, 2:1 ("n")) -> (0:w274:dbl[])
                  n102 = call "Stable.vi"("slope/mean thresh"=w280, "std/mean thresh"=w279, "New data point"=w281, "Number of points"=w278, "Array in"=w282) -> ("Stable?"=w272:bool, "Array out"=w287:dbl[])  [unwired: 5 in]
                  n103 = call "Stable.vi"("slope/mean thresh"=w280, "std/mean thresh"=w279, "New data point"=w277, "Number of points"=w278, "Array in"=w274) -> ("Stable?"=w271:bool, "Array out"=w273:dbl[])  [unwired: 5 in]
                  n104 = local read "Global Stop"() -> (w284:bool)
                  n105 = And(x=w272, y=w271) -> (x .and. y?=w270:bool)
                  n106 = Or(x=w270, y=w284) -> (x .or. y?=w285:bool)
                }
                n107 = case shown="False" w253 {
                  tunnel: w249 -> [w261 w269]
                  tunnel: w252 -> [w262 w268]
                  tunnel: [w259 w267] -> w251
                  tunnel: [w260 w266] -> _
                  tunnel: w235 -> [w263 _]
                  tunnel: 1.5 ("Mask") -> [w258 w264]
                  frame False {
                    n108 = local write "Mask"(w258) -> ()
                    n109 = call "CS580_SetCurent_DC.vi"("error in"=w261, "Current (A)"=w263, "VISA Refnum in"=w262) -> ("error out"=w259:errorcluster, "VISA resource name out"=w260:refnum<visa-resource-name>)  [unwired: 7 in]
                  }
                  frame True {
                    n110 = local write "Mask"(w264) -> ()
                    n111 = call "CS580_SetCurent_DC.vi"("error in"=w269, "Current (A)"=0.001, "VISA Refnum in"=w268) -> ("error out"=w267:errorcluster, "VISA resource name out"=w266:refnum<visa-resource-name>)  [unwired: 7 in]
                  }
                }
                n112 = Multiply(x=w235, y="HTR Guard Current Factor") -> (x*y=w237:dbl)
                n113 = call "setDC.vi"("VISA Refnum in"=w233, "Output Response"=KE6221_--_Output_Response."Slow", "Output State"=KE622x_--_On_Off_Control."On", "Analog Filter State"=KE622x_--_On_Off_Control."Off", "Instrument Type"=KE622x_--_Instrument_Type."KE6221", "Current Level (A)"=w237, "Voltage Limit (V)"=T3 45.0) -> ("error out"=→"Guard Heater Error":errorcluster)  [unwired: 6 in, 2 out]
              }
            }
            n114 = Bundle By Name(cluster=w226, "error out"=w225) -> (w224:T7)
            n115 = local read "Global Stop"() -> (w222:bool)
          }
          frame "Measure (heat)" {
            w306 = Kxx_Kxy_state_machine_cases."Turn off Heater"  # States
            # "WAIT 5 MINS, MEASURE FOR THERMAL CONDUCTIVITY"
            n116 = Unbundle By Name(w296) -> ("HTR Voltage Array"=w305:dbl[], "T_H Array"=w304:dbl[], "T_C1 Array"=w303:dbl[], "T_C2 Array"=w302:dbl[])
            n117 = local read "Calibration Only?"() -> (w307:bool)
            n118 = case shown="False" w307 {
              tunnel: w305 -> [w316 w344]
              tunnel: w304 -> [w313 w343]
              tunnel: w303 -> [w312 w342]
              tunnel: w302 -> [w311 w341]
              tunnel: [w315 w344] -> w301
              tunnel: [w310 w343] -> w300
              tunnel: [w309 w342] -> w299
              tunnel: [w308 w341] -> w298
              frame False {
                w314 = 2.0 ("Mask")
                n119 = local read "Test?"() -> (w318:bool)
                n120 = case shown="True" w318 {
                  tunnel: [300.0 3.0] -> w317
                  tunnel: w314 -> [_ _]
                  frame False {
                  }
                  frame True {
                  }
                }
                n121 = local write "Mask"(w314) -> ()
                n122 = while {
                  shift-right: [w339] -> w310
                  shift-left: w313 -> [w340]
                  shift-right: [w337] -> w308
                  shift-left: w311 -> [w338]
                  shift-right: [w335] -> w315
                  shift-left: w316 -> [w336]
                  shift-right: [w329] -> w309
                  shift-left: w312 -> [w330]
                  tunnel: w317 -> [w325]
                  i -> [w332]
                  stop <- w326 stop-if-true
                  n123 = global read "Thermometers.vi" "Thermometers"() -> (w324:cluster{"T_H":dbl, "T_C1":dbl, "T_C2":dbl})
                  n124 = Wait (ms)(milliseconds to wait=u32 300) -> ()  [unwired: 1 out]
                  n125 = Equal To 0?(x=w332) -> (x = 0?=w331:bool)
                  n126 = Unbundle By Name(w324) -> ("T_H"=w323:dbl, "T_C1"=w322:dbl, "T_C2"=w321:dbl)
                  n127 = call "Elapsed Time6"("Time Target (s)"=w325, "Reset"=w331) -> ("Time has Elapsed"=w328:bool)  [unwired: 10 in, 7 out]
                  n128 = local read "HTR_Voltage"() -> (w334:dbl)
                  n129 = Build Array (concatenate)(w336, w334) -> (w335:dbl[])
                  n130 = Build Array (concatenate)(w340, w323) -> (w339:dbl[])
                  n131 = Build Array (concatenate)(w330, w322) -> (w329:dbl[])
                  n132 = Build Array (concatenate)(w338, w321) -> (w337:dbl[])
                  n133 = local read "Global Stop"() -> (w327:bool)
                  n134 = Or(x=w328, y=w327) -> (x .or. y?=w326:bool)
                }
              }
              frame True {
              }
            }
            n135 = local read "Global Stop"() -> (w294:bool)
            n136 = Bundle By Name(cluster=w296, "HTR Voltage Array"=w301, "T_H Array"=w300, "T_C1 Array"=w299, "T_C2 Array"=w298) -> (w297:T7)
          }
          frame "Turn off Heater" {
            w346 = 2.5 ("Mask")
            w361 = Kxx_Kxy_state_machine_cases."Assign Heater Current"  # States
            # "FIGURE OUT NEW HEATER CURRENT"
            n137 = local read "Calibration Only?"() -> (w363:bool)
            n138 = Unbundle By Name(w356) -> ("HTR Voltage Array"=w360:dbl[], "T_H Array"=w357:dbl[], "T_C1 Array"=w358:dbl[], "T_C2 Array"=w359:dbl[], "error out"=w355:errorcluster)
            n139 = local write "Mask"(w346) -> ()
            n140 = case shown="False" w363 {
              tunnel: w362 -> [w378 _]
              tunnel: w355 -> [w377 w391]
              tunnel: w359 -> [w367 _]
              tunnel: w357 -> [w368 _]
              tunnel: w360 -> [w369 _]
              tunnel: [w385 0.0] -> w352
              tunnel: [w370 0.0] -> w353
              tunnel: [w379 0.0] -> w350
              tunnel: [w376 w391] -> w354
              tunnel: w358 -> [w366 _]
              tunnel: [w372 0.0] -> w351
              tunnel: w346 -> [_ _]
              tunnel: w345 -> [w365 _]
              frame False {
                n141 = call-poly <vilib>:"Mean.vi"("X"=w369) -> ("mean"=w383:dbl)  [unwired: 1 out]
                n142 = call-poly <vilib>:"Mean.vi"("X"=w367) -> ("mean"=w374:dbl)  [unwired: 1 out]
                n143 = local read "HTR_Current"() -> (w384:dbl)
                n144 = VISA Write(VISA resource name=w378, write buffer="SOUT 0", error in (no error)=w377) -> (error out=w376:errorcluster)  [unwired: 2 out]
                n145 = call-poly <vilib>:"Mean.vi"("X"=w366) -> ("mean"=w373:dbl)  [unwired: 1 out]
                n146 = call-poly <vilib>:"Mean.vi"("X"=w368) -> ("mean"=w382:dbl)  [unwired: 1 out]
                n147 = Multiply(x=w384, y=w383) -> (x*y=w371:dbl)
                n148 = Subtract(x=w374, y=w373) -> (x-y=w372:dbl)
                n149 = Subtract(x=w382, y=w374) -> (x-y=w385:dbl)
                n150 = call "KE622x -- Set Output State.vi"("Resource In"=w365, "Output State"=KE622x_--_On_Off_Control."Off") -> ()  [unwired: 12 in, 2 out]
                n151 = Add(x=w382, y=w374) -> (x+y=w381:dbl)
                n152 = Absolute Value(x=w371) -> (abs(x)=w370:dbl)
                n153 = Divide(x=w381, y=2.0) -> (x/y=w379:dbl)
                n154 = Wait (ms)(milliseconds to wait=u32 5000) -> ()  [unwired: 1 out]
              }
              frame True {
              }
            }
            n155 = local read "Global Stop"() -> (w347:bool)
            n156 = Bundle By Name(cluster=w356, "T_avg"=w350, "dTxx"=w352, "dTxy"=w351, "HTR Power"=w353, "error out"=w354) -> (w349:T7)
          }
          frame "Assign Heater Current" {
            n157 = local read "Preset Heater Current Array?"() -> (w398:bool)
            n158 = Unbundle By Name(w396) -> ("dTxx"=w397:dbl)
            n159 = case shown="False" w398 {
              tunnel: w397 -> [w404 _]
              tunnel: w394 -> [_ w417]
              frame False {
                n160 = local read "DeltaT (fraction of tsp)"() -> (w399:dbl)
                n161 = local read "Tsp"() -> (w406:dbl)
                n162 = Multiply(x=w399, y=w406) -> (x*y=w405:dbl)
                n163 = Divide(x=w405, y=w404) -> (x/y=w403:dbl)
                n164 = Square Root(x=w403) -> (sqrt(x)=w402:dbl)
                n165 = Less?(x=w402, y=1.6) -> (x < y?=w400:bool)
                n166 = case shown="True" w400 {
                  tunnel: w402 -> [_ w414]
                  frame False {
                    n167 = local read "HTR_Current"() -> (w408:dbl)
                    n168 = Multiply(x=w408, y=1.3) -> (x*y=w407:dbl)
                    n169 = local write "HTR_Current"(w407) -> ()
                  }
                  frame True {
                    n170 = local read "HTR_Current"() -> (w413:dbl)
                    n171 = Multiply(x=w413, y=w414) -> (x*y=w411:dbl)
                    n172 = Less?(x=w411, y=0.00075) -> (x < y?=w410:bool)
                    n173 = case shown="True" w410 {
                      tunnel: w411 -> [_ w416]
                      frame False {
                        n174 = local write "HTR_Current"(0.00075 ("HTR_Current")) -> ()
                      }
                      frame True {
                        n175 = local write "HTR_Current"(w416) -> ()
                      }
                    }
                  }
                }
              }
              frame True {
                n176 = local write "HTR_Current"(w417) -> ()
              }
            }
            n177 = local read "Global Stop"() -> (w393:bool)
          }
          frame "Plot" {
            w435 = Kxx_Kxy_state_machine_cases."End"  # States
            n178 = local read "Sample_w"() -> (w431:dbl)
            n179 = local read "Sample_Lxx"() -> (w429:dbl)
            n180 = local read "Sample_t"() -> (w430:dbl)
            n181 = local read "Sample_Lxy"() -> (w440:dbl)
            n182 = Unbundle By Name(w434) -> ("T_avg"=w433:dbl, "dTxx"=w432:dbl, "dTxy"=w420:dbl, "HTR Power"=w419:dbl)
            n183 = call "Kxx_Kxy_calc.vi"("Sample_w"=w431, "HTR Power"=w419, "Sample_t"=w430, "dTxy"=w420, "dTxx"=w432, "Sample_Lxx"=w429, "Sample_Lxy"=w440) -> ("Kxx"=w439:dbl, "Kxy"=w438:dbl)  [unwired: 3 in]
            n184 = Unbundle By Name(w425) -> ("T_avg data"=w428:dbl[], "Kxx data"=w427:dbl[], "Kxy data"=w426:dbl[])
            n185 = Build Array (concatenate)(w427, w439) -> (w423:dbl[])
            n186 = Build Array (concatenate)(w426, w438) -> (w422:dbl[])
            n187 = Build Array (concatenate)(w428, w433) -> (w424:dbl[])
            n188 = local read "Calibration Only?"() -> (w436:bool)
            n189 = Bundle(w424, w422) -> (w437:cluster{dbl[], dbl[]})  [unwired: 1 in]
            n190 = Bundle(w424, w423) -> (w441:cluster{dbl[], dbl[]})  [unwired: 1 in]
            n191 = Bundle By Name(cluster=w425, "T_avg data"=w424, "Kxx data"=w423, "Kxy data"=w422) -> (w421:T6)
            n192 = case shown="True" w436 {
              tunnel: w441 -> [_ w443]
              tunnel: w437 -> [_ w442]
              frame True {
              }
              frame False {
                "Kxx Plot" <- w443
                "Kxy Plot" <- w442
              }
            }
            n193 = local read "Global Stop"() -> (w418:bool)
          }
          frame "End" {
          }
        }
        n194 = Wait (ms)(milliseconds to wait=u32 10) -> ()  [unwired: 1 out]
      }
      n195 = local read "Global Stop"() -> (w124:bool)
    }
    n196 = local read "Global Stop"() -> (w99:bool)
    "Fieldsp" <- w119
  }
  n197 = Less?(x="Initial Heater Current (A)", y=0.0004) -> (x < y?=w22:bool)
  n198 = case shown="True" w22 {
    tunnel: "Initial Heater Current (A)" -> [_ w449]
    frame False {
      n199 = local write "HTR_Current"(0.0004 ("HTR_Current")) -> ()
    }
    frame True {
      n200 = local write "HTR_Current"(w449) -> ()
    }
  }
  n201 = call <instrlib>:"Initialize.vi"("Reset (True)"=TRUE, "VISA resource name"="DC Voltmeter") -> ("error out"=w78:errorcluster, "VISA resource name out"=w77:refnum<visa-resource-name>)  [unwired: 8 in]
  n202 = VISA Write(VISA resource name=w77, write buffer="INIT:CONT ON", error in (no error)=w78) -> (VISA resource name out=w36:refnum<visa-resource-name>, error out=w35:errorcluster)  [unwired: 1 out]
  n203 = property on="Name" class="Ring (strict)"("Strings []"=w6) -> ()  [unwired: 2 in, 2 out]
  n204 = Tick Count (ms)() -> (millisecond timer value=w27:u32)
  n205 = case shown="True" "Quick Data Recording" {
    tunnel: w26 -> [_ w453]
    tunnel: "Delay (ms)" -> [_ w451]
    tunnel: w6 -> [_ w450]
    frame False {
    }
    frame True {
      # "SAVE DATA TO FILE"
      n206 = Strip Path(path=w453) -> (stripped path=w457:path, name=w454:string)
      n207 = Concatenate Strings(w454, ".dat") -> (w456:string)
      n208 = Tick Count (ms)() -> (millisecond timer value=w460:u32)
      n209 = Build Path(base path=w457, name or relative path=w456) -> (appended path=w458:path)
      n210 = call-poly <vilib>:"Write To Spreadsheet File.vi"("append to file? (new file:F)"=TRUE, "1D data"=w450, "file path (dialog if empty)"=w458) -> ("new file path (Not A Path if cancelled)"=w452:path)  [unwired: 5 in]
      n211 = while {
        tunnel: w460 -> [w485]
        tunnel: w452 -> [w477]
        tunnel: w451 -> [w476]
        stop <- w461 stop-if-true
        n212 = Wait (ms)(milliseconds to wait=w476) -> ()  [unwired: 1 out]
        n213 = Tick Count (ms)() -> (millisecond timer value=w484:u32)
        n214 = global read "MQM Data Transfer All.vi" "ZI MFLI"() -> (w463:T8)
        n215 = Subtract(x=w484, y=w485) -> (x-y=w483:u32)
        n216 = Unbundle By Name(w463) -> ("Lockin 1 Demod 0.X(V)"=w474:dbl, "Lockin 1 Demod 0.Theta (deg)"=w473:dbl)
        n217 = Unbundle By Name(w463) -> ("Lockin 2 Demod 0.X(V)"=w472:dbl, "Lockin 2 Demod 0.Theta (deg)"=w471:dbl)
        n218 = Unbundle By Name(w463) -> ("Lockin 3 Demod 0.X(V)"=w470:dbl, "Lockin 3 Demod 0.Theta (deg)"=w469:dbl)
        n219 = global read "MQM Data Transfer All.vi" "PPMS"() -> (w462:T9)
        n220 = Unbundle By Name(w462) -> ("Temperature.Temperature (K)"=w482:dbl, "Field.Field (T)"=w481:dbl)
        n221 = local read "HTR_Voltage"() -> (w468:dbl)
        n222 = local read "HTR_Current"() -> (w467:dbl)
        n223 = local read "I_therm"() -> (w464:dbl)
        n224 = local read "Mask"() -> (w466:dbl)
        n225 = local read "Tsp"() -> (w465:dbl)
        n226 = Build Array(w483, w482, w481, w474, w473, w472, w471, w470, w469, w468, w467, w466, w465, w464) -> (w480:dbl[])
        n227 = call "Write To Spreadsheet File (DBL)2.vi"("format (%.3f)"="%_8f", "append to file? (new file:F)"=TRUE, "1D data"=w480, "file path (dialog if empty)"=w477) -> ("error out"=w475:errorcluster)  [unwired: 3 in, 1 out]
        n228 = local read "Global Stop"() -> (w461:bool)
        n229 = call <vilib>:"Clear Errors.vi"("error in (no error)"=w475) -> ()  [unwired: 5 in, 2 out]
      }
    }
  }
  n230 = while {
    tunnel: w27 -> [w536]
    shift-right: [w530] -> _
    shift-left: 0 -> [w535]
    tunnel: w6 -> [w531]
    shift-right: [w526] -> _
    shift-left: dbl[][] [] ("array w/ subset deleted") -> [w527]
    tunnel: "Delay (ms)" -> [w520]
    tunnel: w36 -> [w512]
    tunnel: [w492] -> w19
    shift-right: [w491] -> w9
    shift-left: w35 -> [w509]
    stop <- "Finish" stop-if-true
    # "PLOT DATA BEING RECORDED TO FILE CONTINUOUSLY"
    n231 = Wait (ms)(milliseconds to wait=w520) -> ()  [unwired: 1 out]
    n232 = Tick Count (ms)() -> (millisecond timer value=w537:u32)
    n233 = global read "MQM Data Transfer All.vi" "ZI MFLI"() -> (w494:T8)
    n234 = VISA Write(VISA resource name=w512, write buffer="FETC?", error in (no error)=w509) -> (VISA resource name out=w511:refnum<visa-resource-name>, error out=w508:errorcluster)  [unwired: 1 out]
    n235 = Subtract(x=w537, y=w536) -> (x-y=w530:u32)
    n236 = global read "MQM Data Transfer All.vi" "PPMS"() -> (w493:T9)
    n237 = Subtract(x=w530, y=w535) -> (x-y=→"Data Rate (ms)":u32)
    n238 = Unbundle By Name(w494) -> ("Lockin 3 Demod 0.X(V)"=w497:dbl, "Lockin 3 Demod 0.Theta (deg)"=w496:dbl)
    n239 = Unbundle By Name(w494) -> ("Lockin 2 Demod 0.X(V)"=w502:dbl, "Lockin 2 Demod 0.Theta (deg)"=w523:dbl)
    n240 = Unbundle By Name(w494) -> ("Lockin 1 Demod 0.X(V)"=w500:dbl, "Lockin 1 Demod 0.Theta (deg)"=w499:dbl)
    n241 = Unbundle By Name(w493) -> ("Temperature.Temperature (K)"=w529:dbl, "Field.Field (T)"=w528:dbl)
    n242 = VISA Read(VISA resource name=w511, byte count=u32 1000, error in (no error)=w508) -> (VISA resource name out=w492:refnum<visa-resource-name>, read buffer=w507:string, error out=w491:errorcluster)  [unwired: 1 out]
    n243 = Build Array(w530, w529, w528) -> (w524:dbl[])
    n244 = global read "Thermometers.vi" "Thermometers"() -> (w489:cluster{"T_H":dbl, "T_C1":dbl, "T_C2":dbl})
    "Thermometers" <- w489
    n245 = Match Pattern(string=w507, regular expression="VDC", offset (0)=0) -> (before substring=w504:string)  [unwired: 3 out]
    n246 = Build Array (concatenate)(w524, w500, w499) -> (w522:dbl[])
    n247 = Fract/Exp String To Number(string=w504) -> (number=w503:dbl)  [unwired: 3 in, 1 out]
    n248 = Build Array (concatenate)(w522, w502, w523) -> (w498:dbl[])
    n249 = local read "HTR_Voltage"() -> (w515:dbl)
    n250 = local read "HTR_Current"() -> (w519:dbl)
    n251 = local read "I_therm"() -> (w501:dbl)
    n252 = Unbundle By Name(w489) -> ("T_H"=w488:dbl, "T_C1"=w487:dbl, "T_C2"=w486:dbl)
    n253 = local write "HTR_Voltage"(w503) -> ()
    n254 = Build Array (concatenate)(w498, w497, w496) -> (w495:dbl[])
    n255 = local read "Mask"() -> (w517:dbl)
    n256 = local read "Fieldsp"() -> (w490:dbl)
    n257 = local read "Tsp"() -> (w516:dbl)
    n258 = Build Array (concatenate)(w495, w515, w519, w517, w516, w501, w488, w487, w486, w490) -> (w518:dbl[])
    n259 = Build Array (concatenate)(w527, w518) -> (w521:dbl[][])
    n260 = flat-sequence {
      tunnel: "Display Elements" -> [w550]
      tunnel: [w543] -> w534
      tunnel: w531 -> [w539]
      tunnel: w521 -> [w538]
      tunnel: w534 -> [w597]
      frame #0 {
        n261 = for {
          tunnel: w550 -> [w579] mode=indexing
          shift-right: [w571] -> w549
          shift-left: dbl[] [] -> [w570]
          shift-right: [w572] -> w547
          shift-left: dbl[][] [] -> [w581]
          shift-right: [w577] -> w543
          shift-left: string[] [] -> [w576]
          tunnel: w539 -> [w573]
          tunnel: w538 -> [w574]
          i -> [w575]
          n262 = Unbundle By Name(w579) -> ("X"=w580:bool, "Y"=w583:bool, "Name"=w578:u16)
          n263 = Index Array(array=w574, index (col)=w578) -> (element=w582:dbl[])  [unwired: 1 in]
          n264 = case shown="False" w583 {
            tunnel: w582 -> [_ w589]
            tunnel: w581 -> [w587 w596]
            tunnel: [w587 w595] -> w572
            tunnel: w578 -> [_ w594]
            tunnel: [w588 w592] -> w577
            tunnel: w576 -> [w588 w591]
            tunnel: w573 -> [_ w590]
            frame False {
            }
            frame True {
              n265 = Build Array (concatenate)(w596, w589) -> (w595:dbl[][])
              n266 = Index Array(array=w590, index=w594) -> (element=w593:string)
              n267 = Build Array (concatenate)(w591, w593) -> (w592:string[])
            }
          }
          n268 = case shown="False" w580 {
            tunnel: w578 -> [_ w586]
            tunnel: w575 -> [_ _]
            tunnel: w573 -> [_ w584]
            frame False {
            }
            frame True {
              n269 = Index Array(array=w584, index=w586) -> (element=w585:string)
              n270 = property on="All Data" class="XYGraph (strict)"("XScale.NameLbl.Text"=w585) -> ()  [unwired: 2 in, 2 out]
            }
          }
          n271 = Select(t=w582, s=w580, f=w570) -> (s? t:f=w571:dbl[])
        }
        n272 = for {
          tunnel: w547 -> [w554] mode=indexing
          tunnel: w549 -> [w556]
          tunnel: [w557] -> w548 mode=indexing
          n273 = case shown="0, Default" "Y-Axis" {
            tunnel: w554 -> [w558 w560 w563]
            tunnel: [w558 w559 w562] -> w551
            frame 0, Default {
            }
            frame 1 {
              n274 = Reciprocal(x=w560) -> (1/x=w559:dbl[])
            }
            frame 2 {
              n275 = Absolute Value(x=w563) -> (abs(x)=w561:dbl[])
              n276 = Logarithm Base 10(1:w561) -> (0:w562:dbl[])
            }
          }
          n277 = case shown="0, Default" "X-Axis" {
            tunnel: w556 -> [w564 w566 w569]
            tunnel: [w564 w565 w568] -> w555
            frame 0, Default {
            }
            frame 1 {
              n278 = Reciprocal(x=w566) -> (1/x=w565:dbl[])
            }
            frame 2 {
              n279 = Absolute Value(x=w569) -> (abs(x)=w567:dbl[])
              n280 = Logarithm Base 10(1:w567) -> (0:w568:dbl[])
            }
          }
          n281 = Bundle(w555, w551) -> (w557:cluster{dbl[], dbl[]})  [unwired: 1 in]
        }
        "All Data" <- w548
        n282 = Array Size(array=w547) -> (size(s)=w546:i32[])
        n283 = Index Array(array=w546, index=0) -> (element=w544:i32)
        n284 = property on="All Data" class="XYGraph (strict)"("LegNumRows"=w544) -> ()  [unwired: 2 in, 2 out]
      }
      frame #1 {
        n285 = for {
          tunnel: w597 -> [w598] mode=indexing
          i -> [w599]
          n286 = property on="All Data" class="XYGraph (strict)"("Active Plot"=w599, "Plot.Plot Name"=w598) -> ()  [unwired: 2 in, 2 out]
        }
      }
    }
    n287 = call "Data length guard.vi"("Max length"=20000, "Array"=w521) -> ("array w/ subset deleted"=w526:dbl[][])  [unwired: 9 in]
    "Global Stop" <- "Finish"
  }
  n288 = VISA Write(VISA resource name=w4, write buffer="SOUT 0") -> (VISA resource name out=w3:refnum<visa-resource-name>)  [unwired: 1 in, 2 out]
  n289 = Unbundle By Name(w18) -> ("error out"=w17:errorcluster)
  n290 = VISA Close(VISA resource name=w14, error in (no error)=w11) -> (error out=→"KE6221 error out":errorcluster)
  n291 = VISA Close(VISA resource name=w3) -> ()  [unwired: 1 in, 1 out]
  n292 = call <instrlib>:"SetTemperature.vi"("Rate"=3.0, "Temperature"="Final Temperature (K)", "error in (no error)"=w17, "Instrument Ref In"=w15) -> ("error out"=w32:errorcluster, "Instrument Ref Out"=w33:refnum<k24>)  [unwired: 3 in, 1 out]
  n293 = call <instrlib>:"SetField.vi"("Rate"=100.0, "Field"="Final Field (Oe)", "error in (no error)"=w32, "Instrument Ref In"=w33) -> ("error out"=→"QD error out":errorcluster)  [unwired: 3 in, 2 out]
  n294 = VISA Close(VISA resource name=w19, error in (no error)=w9) -> (error out=→"KE2182 error out":errorcluster)
